vi "AlazarRead - ATS-SDK.vi"(0 "Handle":u32, 1 "Channel":u32(ring)=1 items=["A"=1, "B"=2, "C"=4, "D"=8], 4 "RecordIn":u32=1, 5 "error in (no error)":errorcluster, 6 "Digitizer Settings":T1={"Digitizer delay (us) "=18.666667, "rf points per line"=4000, "lines per plane"=139, "Samp Rate (Hz)"=100000000.0, "Additional dig delay (us)"=0.0, "Voltage Scale"=0.4, "Pre-Looks"=0, "Offset delay (us)"=2.0, "bits A/D"=0, "Avg Num"=1, "DigTimeOut"=5.0, "Rel Dig Delay"=0.0, "Dig Ch"=0, "LeCroyCluster"={"LeCroy Channels"=[TRUE, FALSE, FALSE, FALSE], "LC read pt offset"=0.0, "Sweep Avg"=FALSE}, "Main Digitizer"=enum."NI Digitizer", "Dig Config"=enum."Single channel", "Digitizer ID Cluster"={"Acqiris/Alazar/SP ID"=[], "NI Instr Handles"=[], "LeCroy VISA"="", "GaGe Handle"={"Handle"=0, "Sample size"=0, "Resolution"=0, "Offset"=0, "Channels"=0, "Boards"=0}, "ATS Ref"="ATS9350", "Acqiris Address"=["PCI::INSTR0"], "ADQRef"=refnum, "adq_cu_ptr"=refnum}, "Trigger Settings"={"Trig Source"=1, "Trig Coupling"=0, "Trig Slope"=0, "Level (mV)"=1500.0}, "Bulk Acq"=FALSE, "Bulk Start Indexes"=[], "Data Ref RF"=refnum, "NI ID/Channel"=[], "Total Dig CH"=1, "Xtra Ann Trig delay (us)"=10.0, "Fix Z Delay?"=FALSE, "One Way Transmission?"=FALSE, "Data Ref Log"=refnum} {"Trigger Settings"."Trig Slope" items=["Positive", "Negative"]; "Trigger Settings"."Level (mV)" format="%.2f"; "Trigger Settings"."Trig Coupling" items=["DC 1 MOhm", "AC 1 MOhm", "DC 50 Ohm", "AC 50 Ohm"]; "Trigger Settings"."Trig Source" items=["Chan 1", "External"]; "Rel Dig Delay" format="%.2f"; "DigTimeOut" format="%.2f"; "Avg Num" min=1; "Offset delay (us)" format="%.2f"; "Additional dig delay (us)" format="%.2f"; "Digitizer delay (us)" format="%.2f"}, 7 "ReadSamples":T5) -> (11 "Return Code":u32, 12 "Clock (s)":dbl format="%.2p", 13 "Binary Data":i16[](array[numeric]), 14 "Handle Out":u32, 15 "TimeStamp (s)":dbl format="%.2p", 17 "Voltage Scaling":dbl, 18 "Presize (s)":dbl format="%.2p", 19 "error out":errorcluster)   [LabVIEW 2022 SP3]
doc: "_____AlazarTech, Scope_____\n\nConfigure the capture clock circuitry."
uses:
  ATS_ReadSamples.ctl
  -DigitizerRoutines/DigitizerSettings.ctl
  -DigitizerRoutines/Digitizer.ctl
  -DigitizerRoutines/DigConfig.ctl
  -DigitizerRoutines/DigitizerID.ctl
  C:/Windows/System32/ADQAPI_dotNet_helper.dll
panel:
  out "Waveform Graph":i16[](graph)
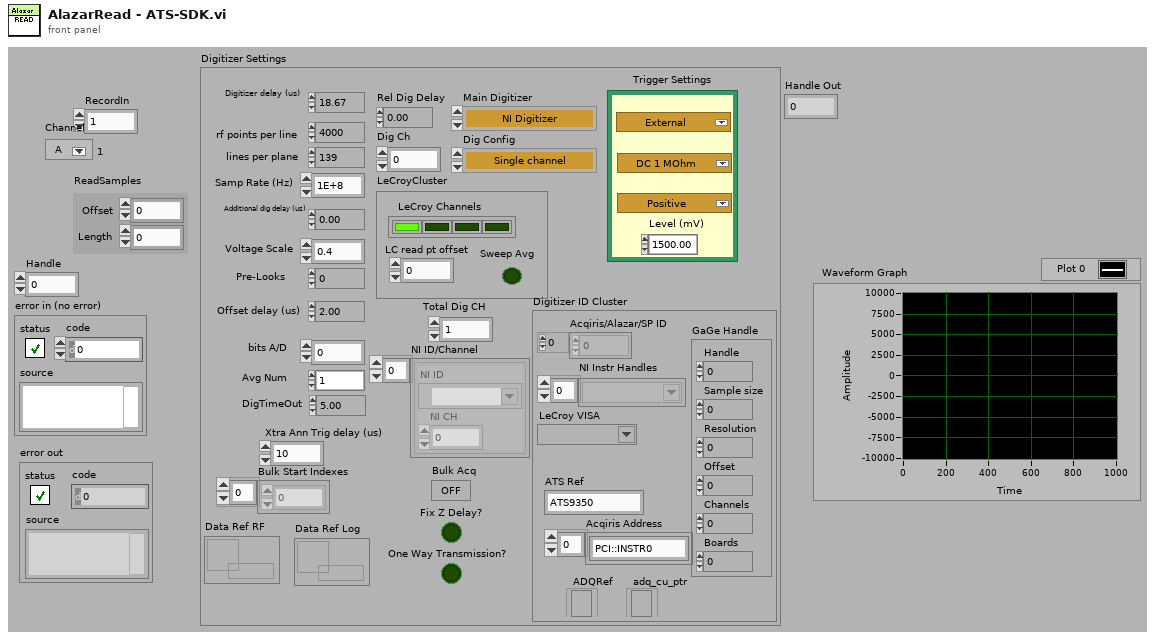
[diagram p1: front panel]
types:
  T1 = typedef "DigitizerSettings.ctl" = cluster{"Digitizer delay (us) ":dbl, "rf points per line":i32, "lines per plane":i32, "Samp Rate (Hz)":dbl, "Additional dig delay (us)":dbl, "Voltage Scale":dbl, "Pre-Looks":i32, "Offset delay (us)":dbl, "bits A/D":i8, "Avg Num":i32, "DigTimeOut":sgl, "Rel Dig Delay":sgl, "Dig Ch":i32, "LeCroyCluster":cluster{"LeCroy Channels":bool[], "LC read pt offset":dbl, "Sweep Avg":bool}, "Main Digitizer":T2, "Dig Config":T3, "Digitizer ID Cluster":T4, "Trigger Settings":cluster{"Trig Source":u16, "Trig Coupling":u16, "Trig Slope":u16, "Level (mV)":dbl}, "Bulk Acq":bool, "Bulk Start Indexes":i32[], "Data Ref RF":refnum<data-value>, "NI ID/Channel":cluster{"NI ID":refnum<k15>, "NI CH":i32}[], "Total Dig CH":i32, "Xtra Ann Trig delay (us)":dbl, "Fix Z Delay?":bool, "One Way Transmission?":bool, "Data Ref Log":refnum<data-value>}
  T2 = typedef "Digitizer.ctl" = enum16{"Acqiris Digitizer", "NI Digitizer", "LeCroy", "GaGe", "AlazarTech", "No Digitizer", "Teledyne"}
  T3 = typedef "DigConfig.ctl" = enum16{"Single channel", "2 Chans w/ 2 Acqiris", "2 Chans w/ 1 Acqiris", "5-CH Pulser New", "5-CH pulser w/ ann array", "5-pass style ann array", "Empty"}
  T4 = typedef "DigitizerID.ctl" = cluster{"Acqiris/Alazar/SP ID":u32[], "NI Instr Handles":refnum<k15>[], "LeCroy VISA":refnum<visa-resource-name>, "GaGe Handle":cluster{"Handle":u32, "Sample size":u32, "Resolution":i32, "Offset":i32, "Channels":u32, "Boards":u32}, "ATS Ref":string, "Acqiris Address":string[], "ADQRef":refnum<k24>, "adq_cu_ptr":refnum<k24>}
  T5 = typedef "ATS_ReadSamples.ctl" = cluster{"Offset":i32, "Length":u32}
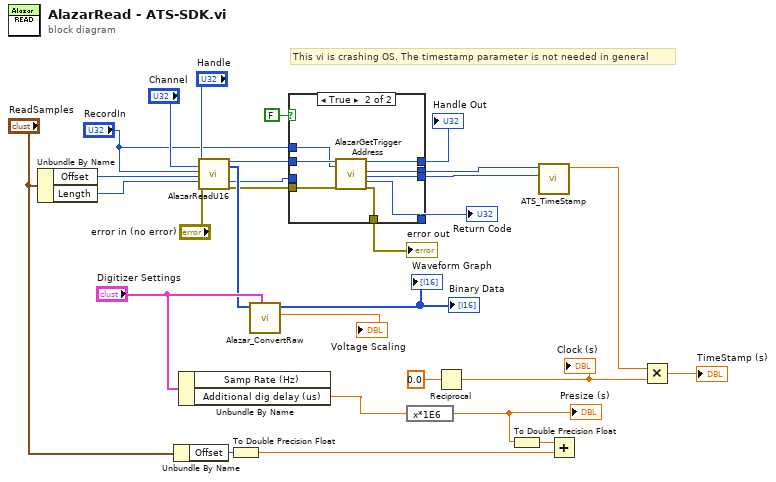
[diagram p0: block diagram]
diagram:
  # "This vi is crashing OS. The timestamp parameter is not needed in general"
  n1 = Unbundle By Name("ReadSamples") -> ("Offset"=w25:i32, "Length"=w24:u32)
  n2 = Unbundle By Name("ReadSamples") -> ("Offset"=w17:i32)
  n3 = Unbundle By Name("Digitizer Settings") -> ("Additional dig delay (us)"=w9:dbl)  [unwired: 1 out]
  n4 = call "AlazarReadU16.vi"("Handle"="Handle", "Channel"="Channel", "Record"="RecordIn", "Transfer Offset"=w25, "Transfer Length"=w24, "error in (no error)"="error in (no error)") -> ("Handle"=w22:u64, "Buffer"=w13:u16[], "Return Code"=w2:u32, "error out"=w11:errorcluster)  [unwired: 10 in]
  n5 = To Double Precision Float(number=w17) -> (double precision float=w16:dbl)
  n6 = call "Alazar_ConvertRaw.vi"("Digitizer Settings"="Digitizer Settings", "Buffer"=w13) -> ("Voltage multiplier"=→"Voltage Scaling":dbl, "Array"=→"Binary Data" →"Waveform Graph":i16[])  [unwired: 8 in]
  n7 = case shown="True" FALSE {
    tunnel: [w32 w40] -> w23
    tunnel: w22 -> [w32 w39]
    tunnel: [w31 w38] -> w21
    tunnel: [w30 w37] -> w20
    tunnel: w11 -> [w30 w36]
    tunnel: "RecordIn" -> [_ w35]
    tunnel: [_ w34] -> w6
    tunnel: [_ w33] -> w5
    tunnel: w2 -> [w31 _]
    frame False {
    }
    frame True {
      n8 = call "AlazarGetTriggerAddress.vi"("Handle"=w39, "Record"=w35, "error in (no error)"=w36) -> ("Handle"=w40:u64, "Timestamp High Part"=w34:u32, "Timestamp Low Part"=w33:u32, "Return Code"=w38:u32, "error out"=w37:errorcluster)  [unwired: 11 in, 1 out]
    }
  }
  "Return Code" <- w21
  "Handle Out" <- w23
  "error out" <- w20
  n9 = expression code="x*1E6"(w9) -> (w8:dbl)
  "Presize (s)" <- w8
  n10 = Reciprocal(x=0.0) -> (1/x=w10:dbl)
  "Clock (s)" <- w10
  n11 = To Double Precision Float(number=w8) -> (double precision float=w18:dbl)
  n12 = call "ATS_TimeStamp.vi"("TimeStampLow"=w5, "TimeStampHigh"=w6) -> ("TimeStamp_Clk"=w4:dbl)  [unwired: 9 in]
  n13 = Add(x=w18, y=w16) -> ()  [unwired: 1 out]
  n14 = Multiply(x=w4, y=w10) -> (x*y=→"TimeStamp (s)":dbl)
